vi "close.vi"(8 "error in (no error)":errorcluster, 11 "rethinkdb in":refnum<class "RethinkDB.lvclass">) -> (0 "error out":errorcluster)   [LabVIEW 2017, in "rethinkdb.lvlib" / "RethinkDB.lvclass"]
uses:
  RethinkDB.lvclass
  RethinkDB.lvclass/RethinkDB.ctl
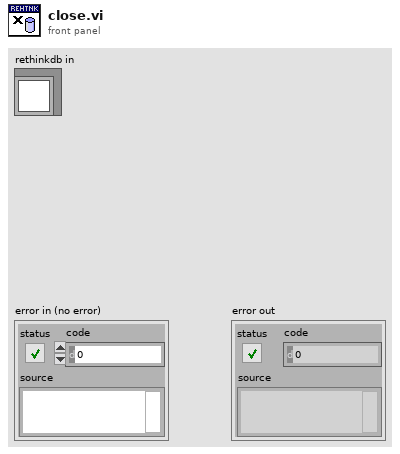
[diagram p1: front panel]
types:
  T1 = typedef "rethinkdb.lvlib/private.ctl" = cluster{"host":string, "port":u16, "ms_timeout":i32, "conn":refnum<k5>, "auth_key":string}
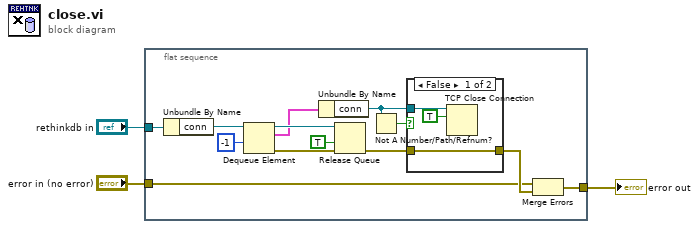
[diagram p0: block diagram]
diagram:
  n1 = flat-sequence {
    tunnel: "rethinkdb in" -> [w11]
    tunnel: [w5] -> w2
    tunnel: "error in (no error)" -> [w4]
    frame #0 {
      n2 = Unbundle By Name(w11) -> ("conn"=w10:refnum<queue>)
      n3 = Dequeue Element(queue=w10, timeout in ms (-1)=-1) -> (queue out=w9:refnum<queue>, element=w6:T1, error out=w8:errorcluster)  [unwired: 1 in, 1 out]
      n4 = Unbundle By Name(w6) -> ("conn"=w15:refnum<k5>)
      n5 = Release Queue(queue=w9, force destroy? (F)=TRUE, error in (no error)=w8) -> (error out=w12:errorcluster)  [unwired: 2 out]
      n6 = Not A Number/Path/Refnum?(number/path/refnum=w15) -> (NaN/Path/Refnum?=w14:bool)
      n7 = case shown="False" w14 {
        tunnel: w15 -> [w19 _]
        tunnel: [w18 w20] -> w13
        tunnel: w12 -> [w18 w20]
        frame False {
          n8 = TCP Close Connection(connection ID=w19, abort (F)=TRUE) -> ()  [unwired: 1 in, 2 out]
        }
        frame True {
        }
      }
      n9 = Merge Errors(w4, w13) -> (w5:errorcluster)
    }
  }
  "error out" <- w2
